vi "2 - Simulate Signal to Graph (Solution).vi"() -> ()   [LabVIEW 2012]
panel:
  in  "Frequency":dbl(knob) scale=0.0..50.0
  in  "Amplitude":dbl(knob) scale=0.0..10.0
  out "Waveform Chart":dynamicdata(graph)
  in  "stop":bool
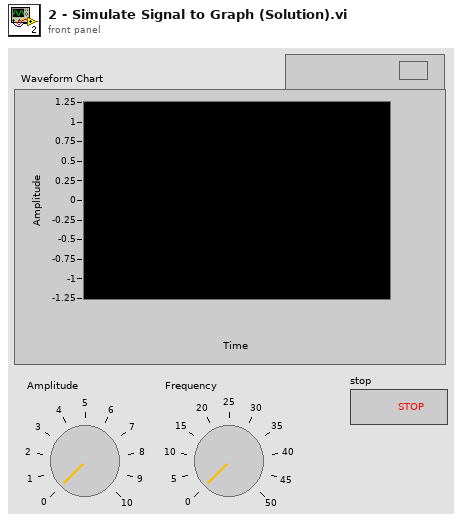
[diagram p1: front panel]
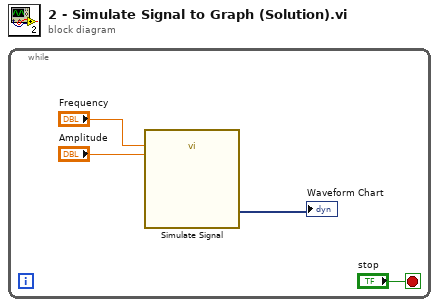
[diagram p0: block diagram]
diagram:
  n1 = while {
    stop <- "stop" stop-if-true
    n2 = call "Simulate Signal"("Frequency"="Frequency", "Amplitude"="Amplitude") -> ("Simulated Signal"=→"Waveform Chart":dynamicdata)  [unwired: 4 in, 9 out]
  }
